vi "niUSRP EX Rx Multiple Inputs (Single Device, Multi Channel).vi"() -> ()   [LabVIEW 2019]
doc: "Configures a single device to use two Rx channels in a synchronous manner."
uses:
  <instrlib>/niUSRP/niUSRP Timestamp.ctl
  <instrlib>/niUSRP/niUSRP Configure Time Start Trigger.vi
  <instrlib>/niUSRP/niUSRP Fetch Rx Data (2D CDB).vi
  <vilib>/measure/maspectr.llb/FFT Power Spectrum for 1 Chan (CDB).vi
  <vilib>/measure/NI_MAPro.lvlib
panel:
  in  "Enabled Channels":string="0,1"
  in  "Channel 3 Gain":dbl=10.0 format="%#_6f"
  in  "Channel 2 Gain":dbl=10.0 format="%#_6f"
  in  "Channel 3\nActive Antenna":string="RX1"
  in  "Channel 2\nActive Antenna":string="RX1"
  in  "Channel 0 Gain":dbl=10.0 format="%#_6f"
  in  "Channel 0 \nActive Antenna":string="RX1"
  in  "Channel 1 Gain":dbl=10.0 format="%#_6f"
  in  "Channel 1\nActive Antenna":string="RX1"
  out "error out":errorcluster
  in  "Tab Control":T1(tab)
  in  "Channel 0 Carrier\n Frequency [Hz]":dbl=2000000000.0 format="%#_6p"
  in  "Channel 1 Carrier\n Frequency [Hz]":dbl=2000000000.0 format="%#_6p"
  in  "Channel 0 Carrier\n Frequency [Hz]":dbl=2000000000.0 format="%#_6p"
  in  "Channel 1 Carrier\n Frequency [Hz]":dbl=2000000000.0 format="%#_6p"
  in  "Channel 3 Carrier\n  Frequency [Hz]":dbl=2000000000.0 format="%#_6p"
  in  "Channel 2 Carrier\n Frequency [Hz]":dbl=2000000000.0 format="%#_6p"
  in  "Carrier Frequency [Hz]":dbl=2000000000.0 format="%#_6p"
  in  "Start Trigger Time":T2={"whole seconds"=1, "fractional seconds"=0.0}
  in  "IQ Rate [S/sec]":dbl=1000000.0 format="%#_6p"
  out "IQ Graph":dbl[][](graph)
  in  "Number of Samples \nPer Fetch":i64=16384
  in  "Timeout":dbl=10.0
  in  "Stop":bool
  out "Actual Rx Timestamp":T2
  out "Baseband Power Spectrum":cluster{"f0":dbl, "df":dbl, "magnitude":dbl[]}[](graph)
  in  "Device Name":refnum<k15>="192.168.10.2"
  # "NI-2945/2955 Controls"
  # "Note that the NI-2900 and NI-2901 use a single LO for both Rx channels"
  # "Time is set to 0 right before calling Initiate"
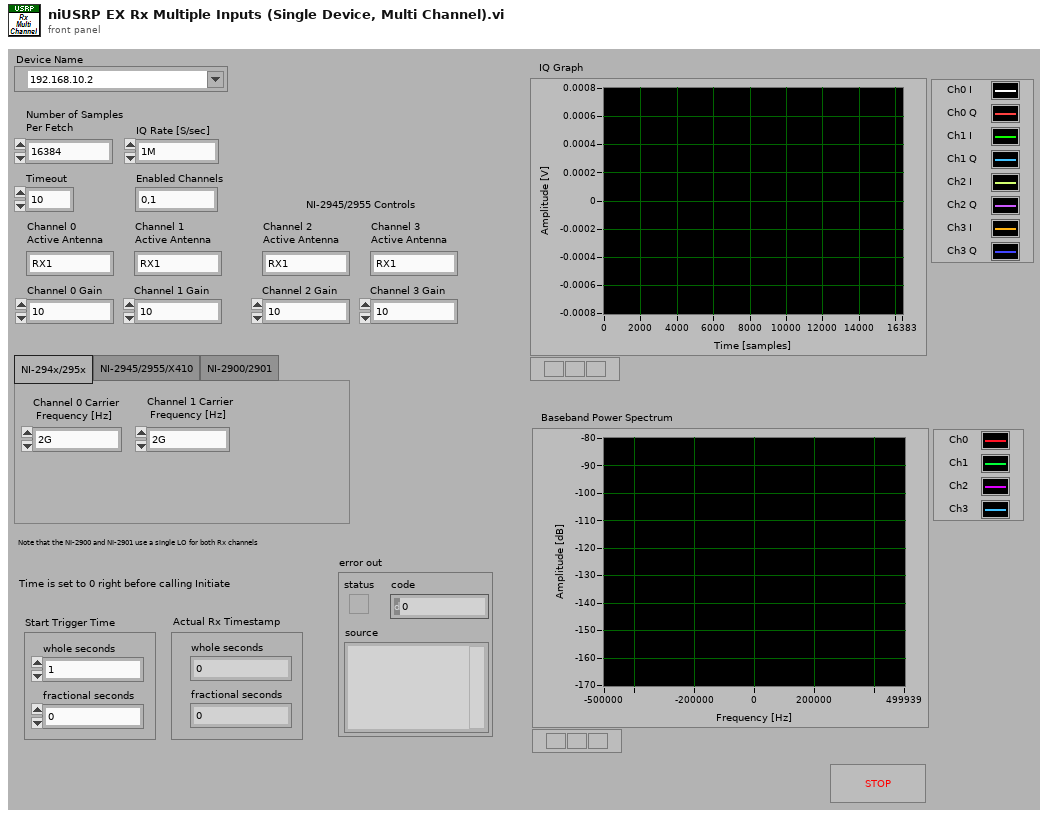
[diagram p1: front panel]
types:
  T1 = enum32{"NI-294x/295x", "NI-2945/2955/X410", "NI-2900/2901"}
  T2 = typedef "niUSRP Timestamp.ctl" = cluster{"whole seconds":u64, "fractional seconds":dbl}
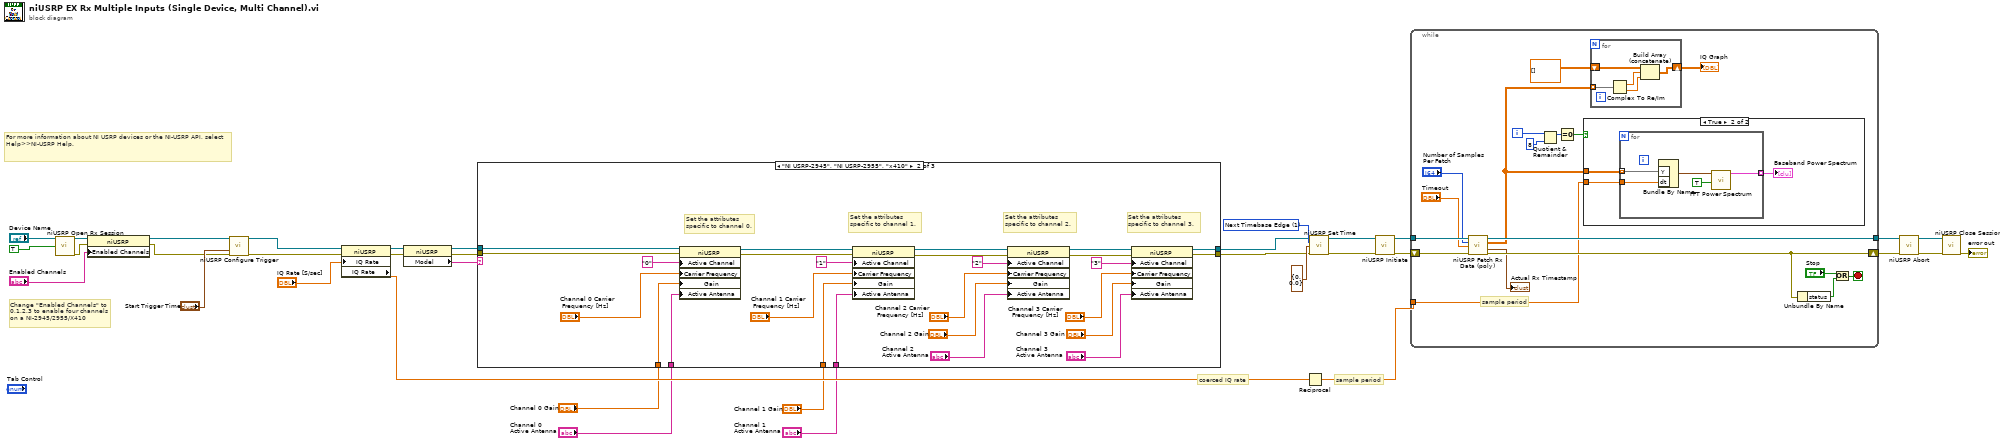
[diagram p0: block diagram]
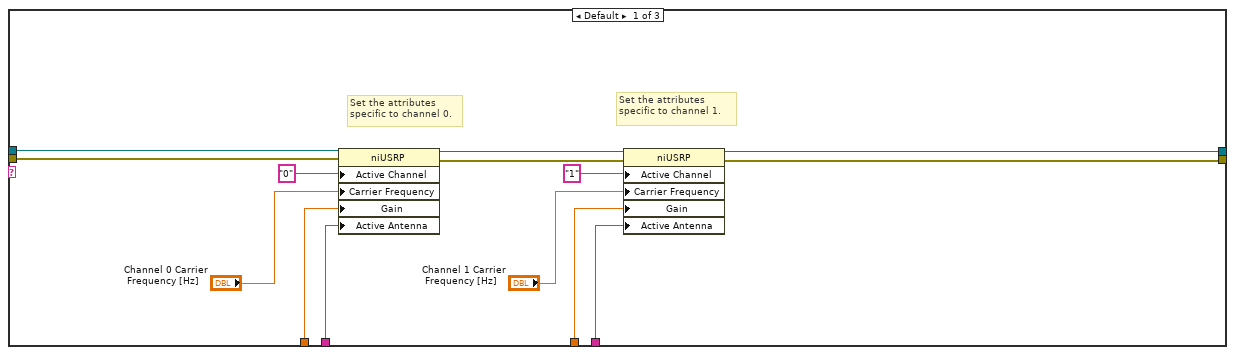
[diagram p2: hidden frame]
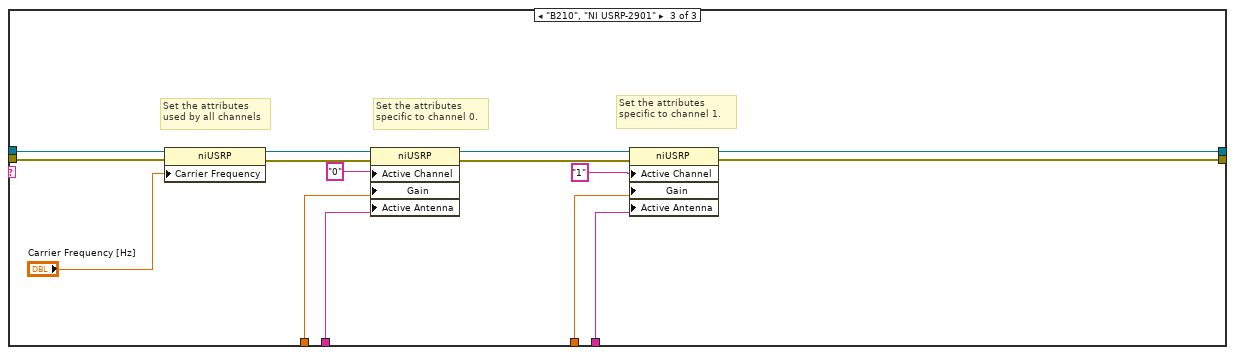
[diagram p3: hidden frame]
diagram:
  w20 = 1 items=["Now", "Next Timebase Edge"] ("apply timestamp")
  # "Change \"Enabled Channels\" to\n0,1,2,3 to enable four channels\non a NI-2945/2955/X410"
  # "For more information about NI USRP devices or the NI-USRP API, select Help>>NI-USRP Help."
  # "sample period"
  # "coerced IQ rate"
  n1 = call <instrlib>:"niUSRP Open Rx Session.vi"("device names"="Device Name", "reset"=TRUE) -> ("session handle out"=w18:refnum<k15>, "error out"=w17:errorcluster)  [unwired: 12 in]
  n2 = property class="niUSRP"(reference=w18, error in=w17, "Enabled Channels"="Enabled Channels") -> (reference out=w16:refnum<k15>, error out=w15:errorcluster)
  n3 = call-poly <instrlib>:"niUSRP Configure Trigger.vi"("session handle"=w16, "start trigger time"="Start Trigger Time", "error in (no error)"=w15) -> ("session handle out"=w14:refnum<k15>, "error out"=w13:errorcluster)  [unwired: 11 in]
  n4 = property class="niUSRP"(reference=w14, error in=w13, "IQ Rate"="IQ Rate [S/sec]") -> (reference out=w9:refnum<k15>, error out=w11:errorcluster, "IQ Rate"=w27:dbl)
  n5 = property class="niUSRP"(reference=w9, error in=w11) -> (reference out=w8:refnum<k15>, error out=w10:errorcluster, "Model"=w12:string)
  n6 = case shown="\"NI USRP-2945\", \"NI USRP-2955\", \"x410\"" w12 {
    tunnel: w10 -> [w45 w71 w80]
    tunnel: w8 -> [w44 w70 w81]
    tunnel: [w43 w63 w86] -> w3
    tunnel: [w42 w62 w76] -> w2
    tunnel: "Channel 0 Gain" -> [w41 w69 w85]
    tunnel: "Channel 0 \nActive Antenna" -> [w40 w68 w84]
    tunnel: "Channel 1 Gain" -> [w39 w67 w83]
    tunnel: "Channel 1\nActive Antenna" -> [w38 w66 w82]
    frame Default {
      # "Set the attributes \nspecific to channel 1."
      # "Set the attributes \nspecific to channel 0."
      n7 = property class="niUSRP"(reference=w44, error in=w45, "Active Channel"="0", "Carrier Frequency"="Channel 0 Carrier\n Frequency [Hz]", "Gain"=w41, "Active Antenna"=w40) -> (reference out=w49:refnum<k15>, error out=w48:errorcluster)
      n8 = property class="niUSRP"(reference=w49, error in=w48, "Active Channel"="1", "Carrier Frequency"="Channel 1 Carrier\n Frequency [Hz]", "Gain"=w39, "Active Antenna"=w38) -> (reference out=w43:refnum<k15>, error out=w42:errorcluster)
    }
    frame "NI USRP-2945", "NI USRP-2955", "x410" {
      # "Set the attributes \nspecific to channel 3."
      # "Set the attributes \nspecific to channel 2."
      # "Set the attributes \nspecific to channel 1."
      # "Set the attributes \nspecific to channel 0."
      n9 = property class="niUSRP"(reference=w70, error in=w71, "Active Channel"="0", "Carrier Frequency"="Channel 0 Carrier\n Frequency [Hz]", "Gain"=w69, "Active Antenna"=w68) -> (reference out=w75:refnum<k15>, error out=w74:errorcluster)
      n10 = property class="niUSRP"(reference=w75, error in=w74, "Active Channel"="1", "Carrier Frequency"="Channel 1 Carrier\n Frequency [Hz]", "Gain"=w67, "Active Antenna"=w66) -> (reference out=w65:refnum<k15>, error out=w60:errorcluster)
      n11 = property class="niUSRP"(reference=w65, error in=w60, "Active Channel"="2", "Carrier Frequency"="Channel 2 Carrier\n Frequency [Hz]", "Gain"="Channel 2 Gain", "Active Antenna"="Channel 2\nActive Antenna") -> (reference out=w64:refnum<k15>, error out=w61:errorcluster)
      n12 = property class="niUSRP"(reference=w64, error in=w61, "Active Channel"="3", "Carrier Frequency"="Channel 3 Carrier\n  Frequency [Hz]", "Gain"="Channel 3 Gain", "Active Antenna"="Channel 3\nActive Antenna") -> (reference out=w63:refnum<k15>, error out=w62:errorcluster)
    }
    frame "B210", "NI USRP-2901" {
      # "Set the attributes \nused by all channels"
      # "Set the attributes \nspecific to channel 1."
      # "Set the attributes \nspecific to channel 0."
      n13 = property class="niUSRP"(reference=w81, error in=w80, "Carrier Frequency"="Carrier Frequency [Hz]") -> (reference out=w79:refnum<k15>, error out=w78:errorcluster)
      n14 = property class="niUSRP"(reference=w79, error in=w78, "Active Channel"="0", "Gain"=w85, "Active Antenna"=w84) -> (reference out=w90:refnum<k15>, error out=w89:errorcluster)
      n15 = property class="niUSRP"(reference=w90, error in=w89, "Active Channel"="1", "Gain"=w83, "Active Antenna"=w82) -> (reference out=w86:refnum<k15>, error out=w76:errorcluster)
    }
  }
  n16 = Reciprocal(x=w27) -> (1/x=w26:dbl)
  n17 = call <instrlib>:"niUSRP Set Time.vi"("session handle"=w3, "apply timestamp"=w20, "timestamp"=T2 {"whole seconds"=0, "fractional seconds"=0.0}, "error in (no error)"=w2) -> ("session handle out"=w22:refnum<k15>, "error out"=w21:errorcluster)  [unwired: 10 in]
  n18 = call <instrlib>:"niUSRP Initiate.vi"("session handle"=w22, "error in (no error)"=w21) -> ("session handle out"=w35:refnum<k15>, "error out"=w34:errorcluster)  [unwired: 12 in]
  n19 = while {
    tunnel: w35 -> [w108]
    tunnel: [w104] -> w33
    shift-right: [w103] -> w32
    shift-left: w34 -> [w107]
    tunnel: w26 -> [w91]
    i -> [w95]
    stop <- w102 stop-if-true
    # "sample period"
    n20 = call-poly <instrlib>:"niUSRP Fetch Rx Data (poly).vi"("session handle"=w108, "number of samples"="Number of Samples \nPer Fetch", "timeout"="Timeout", "error in (no error)"=w107) -> ("session handle out"=w104:refnum<k15>, "data"=w92:cdb[][], "timestamp"=→"Actual Rx Timestamp":T2, "error out"=w103:errorcluster)  [unwired: 8 in]
    n21 = Quotient & Remainder(x=w95, y=8) -> (x-y*floor(x/y)=w96:i32)  [unwired: 1 out]
    n22 = Equal To 0?(x=w96) -> (x = 0?=w93:bool)
    n23 = case shown="True" w93 {
      tunnel: w92 -> [_ w110]
      tunnel: w91 -> [_ w109]
      frame False {
      }
      frame True {
        n24 = for {
          tunnel: [w116] -> w111 mode=indexing
          tunnel: w110 -> [w114] mode=indexing
          tunnel: w109 -> [w112]
          n25 = Bundle By Name("Y"=w114, "dt"=w112) -> (w113:waveform(cdb))  [unwired: 1 in]
          n26 = call-poly <vilib>:"FFT Power Spectrum.vi"("dB On (F)"=TRUE, "time signal"=w113) -> ("power spectrum"=w116:cluster{"f0":dbl, "df":dbl, "magnitude":dbl[]})  [unwired: 6 in, 3 out]
        }
        "Baseband Power Spectrum" <- w111
      }
    }
    n27 = for {
      tunnel: w92 -> [w121] mode=indexing
      shift-right: [w118] -> w97
      shift-left: dbl[][] [] -> [w117]
      n28 = Complex To Re/Im(x + iy=w121) -> (x=w120:dbl[], y=w119:dbl[])
      n29 = Build Array (concatenate)(w117, w120, w119) -> (w118:dbl[][])
    }
    "IQ Graph" <- w97
    n30 = Unbundle By Name(w103) -> ("status"=w99:bool)
    n31 = Or(x="Stop", y=w99) -> (x .or. y?=w102:bool)
  }
  n32 = call <instrlib>:"niUSRP Abort.vi"("session handle"=w33, "error in (no error)"=w32) -> ("session handle out"=w30:refnum<k15>, "error out"=w31:errorcluster)  [unwired: 12 in]
  n33 = call <instrlib>:"niUSRP Close Session.vi"("session handle"=w30, "error in (no error)"=w31) -> ("error out"=→"error out":errorcluster)  [unwired: 13 in]
